vi "ingest.video.vi"(8 "error in":errorcluster, 11 "Client in":refnum<class "Client.lvclass">) -> (0 "error out":errorcluster, 3 "Client out":refnum<class "Client.lvclass">)   [LabVIEW 2020, in "Client.lvclass"]
doc: "Ingests a standalone video file into an existing video resource, given its start time."
uses:
  Client.lvclass
  Client.lvclass/Client.ctl
  client.lvlib
panel:
  out "out_job out":i32
  in  "file_path":string
  in  "video_rid":string
  in  "start_ms":dbl
  in  "out_job":i32
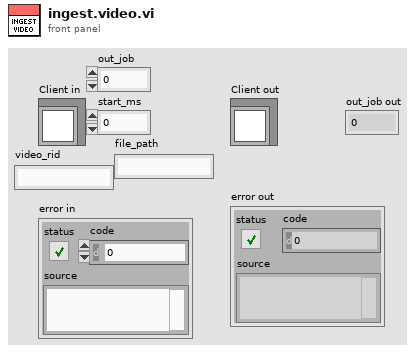
[diagram p1: front panel]
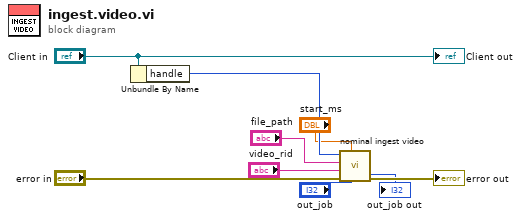
[diagram p0: block diagram]
diagram:
  n1 = Unbundle By Name("Client in") -> ("handle"=w7:i32)
  n2 = call "nominal ingest video.vi"("out_job"="out_job", "start_ms"="start_ms", "error in (no error)"="error in", "video_rid"="video_rid", "file_path"="file_path", "client"=w7) -> ("error out"=→"error out":errorcluster, "out_job out"=→"out_job out":i32)  [unwired: 3 in, 1 out]
  "Client out" <- "Client in"
